vi "Untitled 6.vi"() -> ()   [LabVIEW 2018]
uses:
  <userlib>/stepper/velocity settings.ctl
  <userlib>/stepper/travel limits.ctl
panel:
  in  "Slide":dbl(slide) scale=0.0..4.5
  out "travel limits":T1
  out "velocity parameters":T2
  out "Waveform Chart":sgl(graph)
  out "pfPosition":sgl
  in  "stop":bool
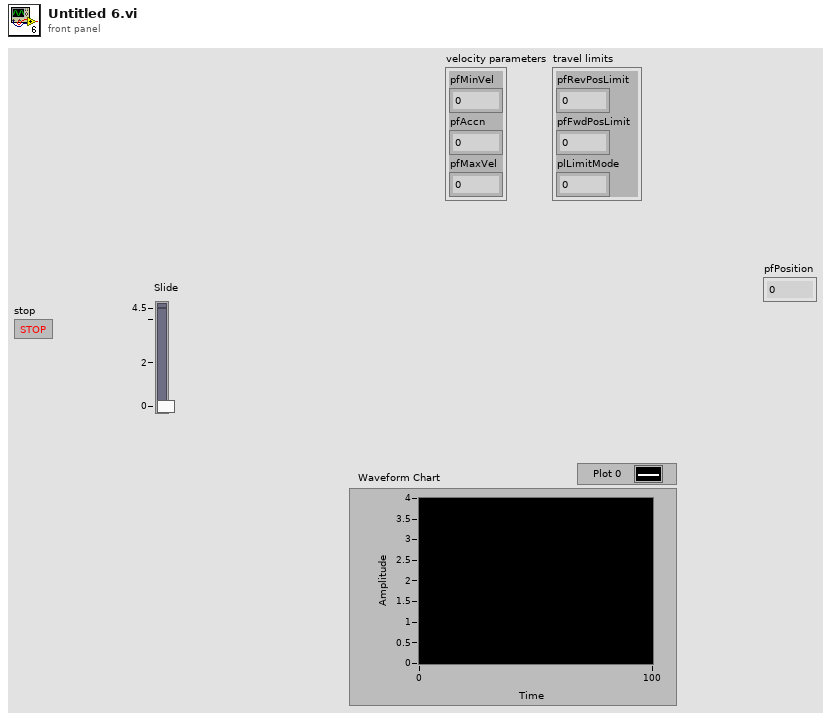
[diagram p1: front panel]
types:
  T1 = cluster{"pfRevPosLimit":sgl, "pfFwdPosLimit":sgl, "plLimitMode":i32}
  T2 = cluster{"pfMinVel":sgl, "pfAccn":sgl, "pfMaxVel":sgl}
  T3 = typedef "travel limits.ctl" = cluster{"pfRevPosLimit":sgl, "pfFwdPosLimit":sgl, "plLimitMode":i32}
  T4 = typedef "velocity settings.ctl" = cluster{"pfMinVel":sgl, "pfAccn":sgl, "pfMaxVel":sgl}
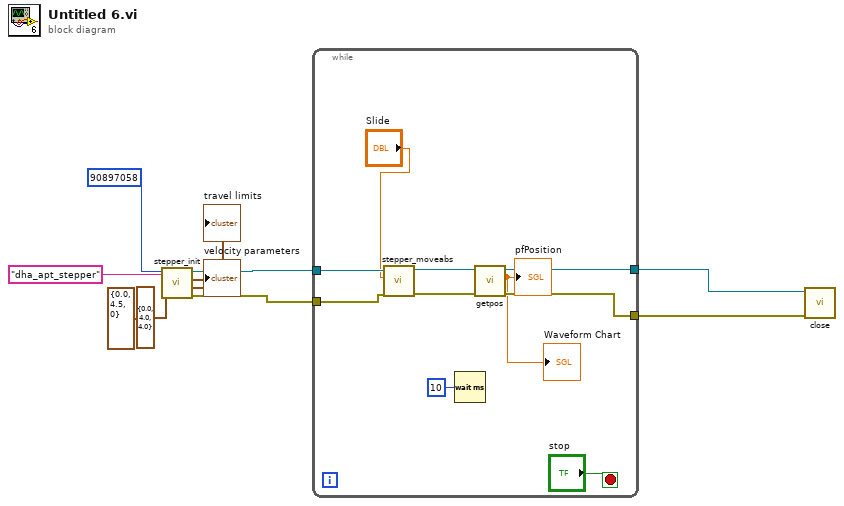
[diagram p0: block diagram]
diagram:
  n1 = call <userlib>:"stepper_init.vi"("travel limits"=T3 {"pfRevPosLimit"=0.0, "pfFwdPosLimit"=4.5, "plLimitMode"=0}, "velocity parameters"=T4 {"pfMinVel"=0.0, "pfAccn"=4.0, "pfMaxVel"=4.0}, "parameter set"="dha_apt_stepper", "HWSerialNum"=90897058) -> ("error out"=w8:errorcluster, "travel limits"=→"travel limits":T1, "velocity parameters"=→"velocity parameters":T2, "reference out"=w9:refnum<k7>)  [unwired: 4 in]
  n2 = while {
    tunnel: w9 -> [w20]
    tunnel: w8 -> [w19]
    tunnel: [w15] -> w7
    tunnel: [w14] -> w6
    stop <- "stop" stop-if-true
    n3 = call <userlib>:"stepper_moveabs.vi"("error in (no error)"=w19, "fAbsPos"="Slide", "reference"=w20) -> ("error out"=w16:errorcluster, "reference out"=w17:refnum<k7>)  [unwired: 7 in]
    n4 = Wait (ms)(milliseconds to wait=u32 10) -> ()  [unwired: 1 out]
    n5 = call <userlib>:"getpos.vi"("error in (no error)"=w16, "reference"=w17) -> ("error out"=w15:errorcluster, "pfPosition"=→"pfPosition" →"Waveform Chart":sgl, "reference out"=w14:refnum<k7>)  [unwired: 7 in]
  }
  n6 = call <userlib>:"close.vi"("error in (no error)"=w7, "reference"=w6) -> ()  [unwired: 8 in, 2 out]
